vi "Actor Core.vi"(8 "error in":errorcluster, 11 "Report Generator in":refnum<class "Report Generator.lvclass">) -> (0 "error out":errorcluster, 3 "Actor out":refnum<class "Actor.lvclass">)   [LabVIEW 2019, in "Report Generator.lvlib" / "Report Generator.lvclass"]
doc: "The user interface for this panel.\n\n----\nPlease see the following web address for additional documentation and tutorial information:\nhttp://www.mooregoodideas.com/mgi-panel-manager/\n\nAuthor: Derek Trepanier\n\nCopyright (c) 2018, Moore Good Ideas, Inc.\n\nAll rights reserved.\n\nRedistribution and use in source and binary forms, with or without modification, are permitted provided that the following conditions are met:\n\n * Redistributions of source code must retain the above copyright notice, this list of conditions and the following disclaimer.\n * Redistributions in binary form must reproduce the above copyright notice, this list of conditions and the following disclaimer in the documentation and/or other materials provided with the distribution.\n * Neither the name of Moore Good Ideas, Inc. nor the names of its contributors may be used to endorse or promote products derived from this software without specific prior written permission.\n\nTHIS SOFTWARE IS PROVIDED BY THE COPYRIGHT HOLDERS AND CONTRIBUTORS \"AS IS\" AND ANY EXPRESS OR IMPLIED WARRANTIES, INCLUDING, BUT NOT LIMITED TO, THE IMPLIED WARRANTIES OF MERCHANTABILITY AND FITNESS FOR A PARTICULAR PURPOSE ARE DISCLAIMED. IN NO EVENT SHALL THE COPYRIGHT OWNER OR CONTRIBUTORS BE LIABLE FOR ANY DIRECT, INDIRECT, INCIDENTAL, SPECIAL, EXEMPLARY, OR CONSEQUENTIAL DAMAGES (INCLUDING, BUT NOT LIMITED TO, PROCUREMENT OF SUBSTITUTE GOODS OR SERVICES; LOSS OF USE, DATA, OR PROFITS; OR BUSINESS INTERRUPTION) HOWEVER CAUSED AND ON ANY THEORY OF LIABILITY, WHETHER IN CONTRACT, STRICT LIABILITY, OR TORT (INCLUDING NEGLIGENCE OR OTHERWISE) ARISING IN ANY WAY OUT OF THE USE OF THIS SOFTWARE, EVEN IF ADVISED OF THE POSSIBILITY OF SUCH DAMAGE."
uses:
  Library/Report Generator.lvclass
  builds/Engine/Actor Framework.lvlibp/1abvi3w/vi.lib/ActorFramework/Actor/Actor.lvclass
  Library/Report Generator.lvclass/Report Generator.ctl
  builds/Base Software/Panels/Left Panel.lvlibp/Project/Left.lvclass
  builds/Engine/Engine.lvlibp/Project/Engine.lvclass
  C:/Users/Public/Documents/Development/builds/Engine/Engine.lvlibp/Project/Engine.lvclass
panel:
  in  "TestName":string
  in  "Witness":string
  in  "Tester":string
  in  "UUT":string
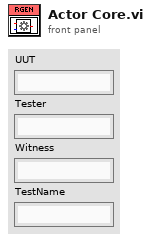
[diagram p1: front panel]
types:
  T1 = cluster{"Pnl Actor":refnum<event-registration>, "Event Registration Refnum":refnum<event-registration>}
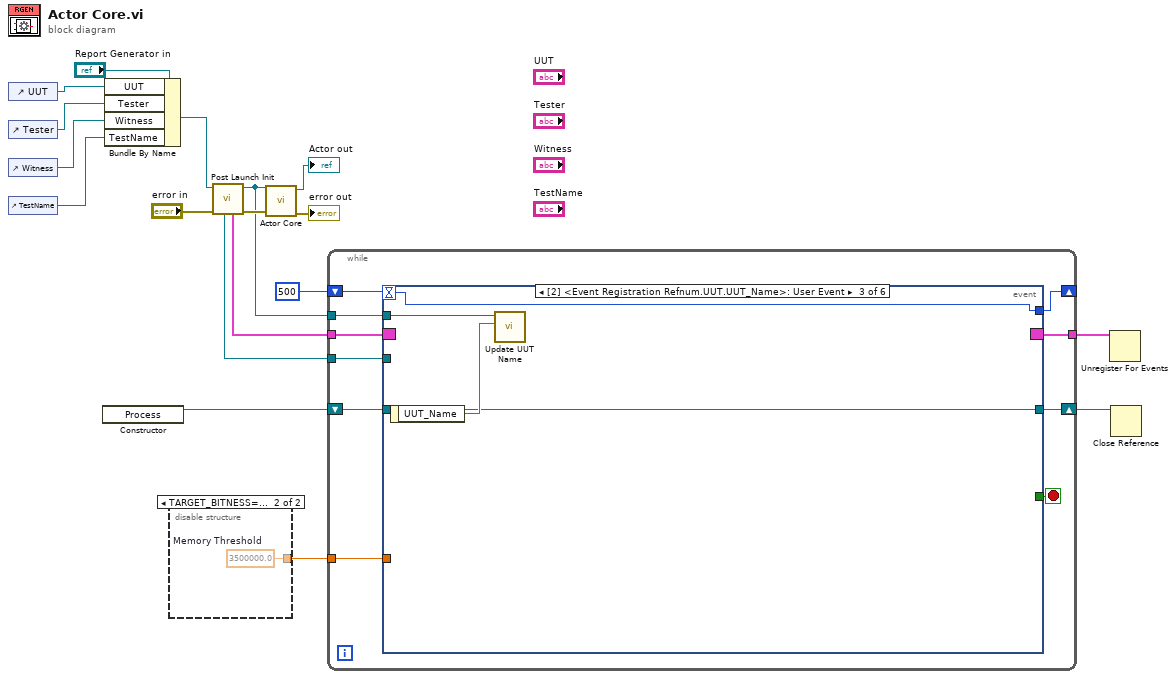
[diagram p0: block diagram]
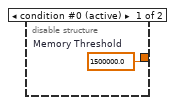
[diagram p2: hidden frame]
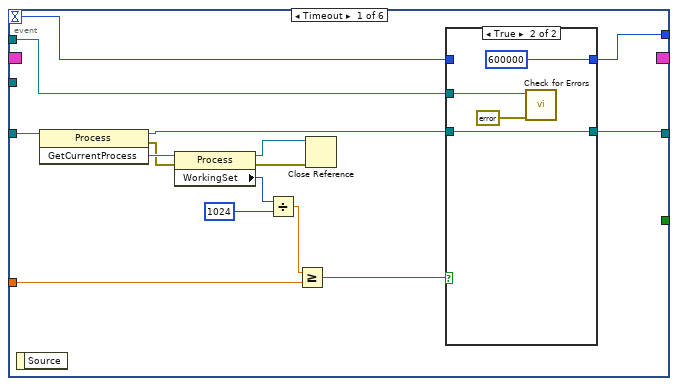
[diagram p3: hidden frame]
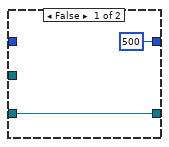
[diagram p4: hidden frame]
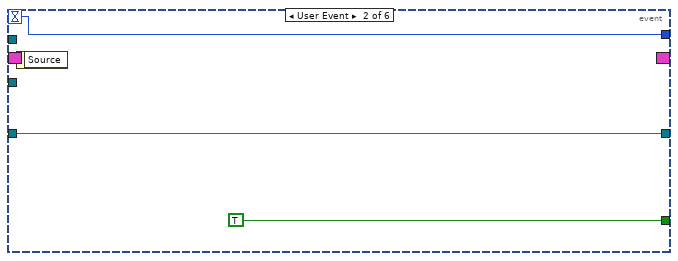
[diagram p5: hidden frame]
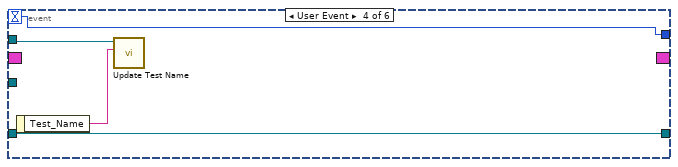
[diagram p6: hidden frame]
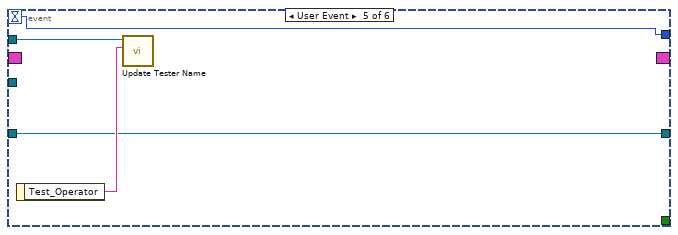
[diagram p7: hidden frame]
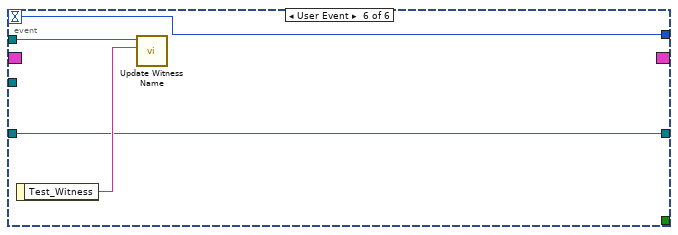
[diagram p8: hidden frame]
diagram:
  n1 = control-ref of="UUT"() -> (w8:refnum<vi>)
  n2 = control-ref of="Tester"() -> (w7:refnum<vi>)
  n3 = control-ref of="Witness"() -> (w6:refnum<vi>)
  n4 = control-ref of="TestName"() -> (w5:refnum<vi>)
  n5 = constructor class="Process"() -> (reference out=w4:refnum<k24>)  [unwired: 3 in, 2 out]
  n6 = Bundle By Name(cluster="Report Generator in", "UUT"=w8, "Tester"=w7, "Witness"=w6, "TestName"=w5) -> (w9:refnum<class "Report Generator.lvclass">)
  n7 = disable-structure shown="TARGET_BITNESS==64" {
    disable-tunnel: [w19 w20] -> w1
    frame condition #0 (active) {
      w19 = 1500000.0  # Memory Threshold
    }
    frame condition #1 {
      w20 = 3500000.0  # Memory Threshold
    }
  }
  n8 = call "Post Launch Init.vi"("error in"="error in", "Report Generator in"=w9) -> ("error out"=w15:errorcluster, "Report Generator out"=w10:refnum<class "Report Generator.lvclass">, "Events"=w12:T1, "Self Enqueuer"=w11:refnum<class "Message Enqueuer.lvclass">)  [unwired: 6 in]
  n9 = call-parent "Actor Core.vi"("error in"=w15, "Left in"=w10) -> ("error out"=→"error out":errorcluster, "Actor out"=→"Actor out":refnum<class "Actor.lvclass">)  [unwired: 8 in]
  n10 = while {
    tunnel: w12 -> [w30]
    tunnel: w11 -> [w29]
    tunnel: [w27] -> w16
    tunnel: w10 -> [w26]
    shift-right: [w24] -> w3
    shift-left: w4 -> [w25]
    shift-right: [w22] -> _
    shift-left: 500 -> [w23]
    tunnel: w1 -> [w21]
    stop <- w28 stop-if-true
    n11 = event shown="[2] <Event Registration Refnum.UUT.UUT_Name>: User Event" {
      selector: w30 -> [_ _ _ _ _ _]
      dyn-events: [_ _ _ _ _ _] -> w27
      timeout: w23 -> [w36 w52 w55 w59 w63 w67]
      tunnel: w29 -> [_ _ _ _ _ _]
      tunnel: [_ TRUE _ _ _ _] -> w28
      tunnel: w26 -> [w31 _ w58 w62 w66 w70]
      tunnel: w25 -> [w45 w53 w56 w60 w64 w68]
      tunnel: [w32 w53 w56 w60 w64 w68] -> w24
      tunnel: [w35 w52 w55 w59 w63 w67] -> w22
      tunnel: w21 -> [w34 _ _ _ _ _]
      event Timeout {
        n12 = event-data() -> ()  [unwired: 1 in, 1 out]
        n13 = invoke class="Process" method="GetCurrentProcess"(reference=w45) -> (reference out=w33:refnum<k24>, error out=w40:errorcluster, "GetCurrentProcess"=w44:refnum<k24>)  [unwired: 2 in]
        n14 = property class="Process"(reference=w44, error in=w40) -> (reference out=w41:refnum<k24>, error out=w39:errorcluster, "WorkingSet"=w43:i32)
        n15 = Divide(x=w43, y=1024) -> (x/y=w38:dbl)
        n16 = Greater Or Equal?(x=w38, y=w34) -> (x >= y?=w37:bool)
        n17 = Close Reference(reference=w41, error in (no error)=w39) -> ()  [unwired: 1 out]
        n18 = case shown="True" w37 {
          tunnel: w36 -> [_ _]
          tunnel: [500 600000] -> w35
          tunnel: w33 -> [w46 w50]
          tunnel: [w46 w50] -> w32
          tunnel: w31 -> [_ w49]
          frame False {
          }
          frame True {
            n19 = call "Check for Errors.vi"("error in"=errorcluster {"status"=FALSE, "code"=5050, "source"="Warning! System Memory Low.  Please Restart the Software."}, "Engine in"=w49) -> ()  [unwired: 8 in, 2 out]
          }
        }
      }
      event User Event {
        n20 = event-data() -> ()  [unwired: 1 in, 1 out]
      }
      event User Event {
        n21 = event-data() -> ("UUT_Name"=w57:string)  [unwired: 1 in]
        n22 = call "Update UUT Name.vi"("UUT_Name"=w57, "Report Generator in"=w58) -> ()  [unwired: 8 in, 2 out]
      }
      event User Event {
        n23 = event-data() -> ("Test_Name"=w61:string)  [unwired: 1 in]
        n24 = call "Update Test Name.vi"("Test_Name"=w61, "Report Generator in"=w62) -> ()  [unwired: 8 in, 2 out]
      }
      event User Event {
        n25 = event-data() -> ("Test_Operator"=w65:string)  [unwired: 1 in]
        n26 = call "Update Tester Name.vi"("Tester_Name"=w65, "Report Generator in"=w66) -> ()  [unwired: 8 in, 2 out]
      }
      event User Event {
        n27 = event-data() -> ("Test_Witness"=w69:string)  [unwired: 1 in]
        n28 = call "Update Witness Name.vi"("Witness_Name"=w69, "Report Generator in"=w70) -> ()  [unwired: 8 in, 2 out]
      }
    }
  }
  n29 = Unregister For Events(event registration refnum=w16) -> ()  [unwired: 1 in, 1 out]
  n30 = Close Reference(reference=w3) -> ()  [unwired: 1 in, 1 out]
